vi "Create Control Custom Device.vi"(8 "error in (no error)":errorcluster, 9 "CD Config Path (.dat)":path, 10 "Name":string, 11 "Custom Devices Ref":refnum<k24>) -> (0 "error out":errorcluster, 3 "Custom Devices Ref":refnum<k24>)   [LabVIEW 2019, in "Control System Definition API.lvlib"]
uses:
  Control System Definition API.lvlib
  NationalInstruments.VeriStand.SystemDefinitionAPI
  Shared/Constants.vi
  <vilib>/NI/NI VeriStand Custom Device Import and Export Tool/ImportExport.lvlib
  Shared/Control Addon Shared.lvlib
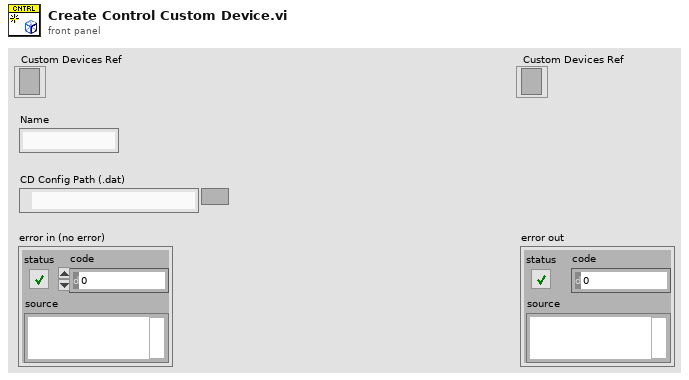
[diagram p1: front panel]
types:
  T1 = typedef "Custom Device API.lvlib/Custom Device Item Ref.ctl" = u64
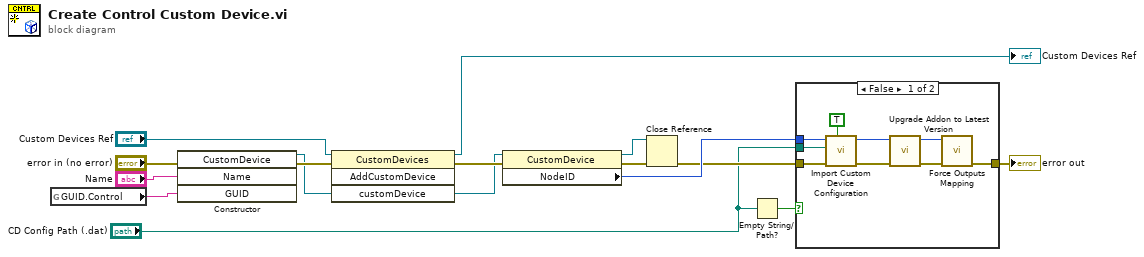
[diagram p0: block diagram]
diagram:
  n1 = global read "Constants.vi" "GUID.Control"() -> (w2:string)
  n2 = constructor class="CustomDevice"(error in="error in (no error)", "Name"="Name", "GUID"=w2) -> (reference out=w8:refnum<k24>, error out=w10:errorcluster)  [unwired: 2 in, 3 out]
  n3 = invoke class="CustomDevices" method="AddCustomDevice"(reference="Custom Devices Ref", error in=w10, "customDevice"=w8) -> (reference out=→"Custom Devices Ref":refnum<k24>, error out=w9:errorcluster)  [unwired: 1 in, 2 out]
  n4 = property class="CustomDevice"(reference=w8, error in=w9) -> (reference out=w7:refnum<k24>, error out=w6:errorcluster, "NodeID"=w13:u64)
  n5 = Close Reference(reference=w7, error in (no error)=w6) -> (error out=w5:errorcluster)
  n6 = Empty String/Path?(string/path="CD Config Path (.dat)") -> (empty?=w3:bool)
  n7 = case shown="False" w3 {
    tunnel: w13 -> [w24 _]
    tunnel: [w17 w25] -> w12
    tunnel: w5 -> [w22 w25]
    tunnel: "CD Config Path (.dat)" -> [w21 _]
    frame False {
      n8 = call <vilib>:"Import Custom Device Configuration.vi"("Overwrite Existing?"=TRUE, "error in (no error)"=w22, "Path"=w21, "NodeID"=w24) -> ("error out"=w20:errorcluster, "NodeID out"=w19:u64)  [unwired: 5 in, 1 out]
      n9 = call "Upgrade Addon to Latest Version.vi"("error in (no error)"=w20, "Device Item Ref in in"=w19) -> ("error out"=w16:errorcluster, "Device Item Ref out"=w18:T1)  [unwired: 8 in]
      n10 = call "Force Outputs Mapping.vi"("error in (no error)"=w16, "Device Item Ref in"=w18) -> ("error out"=w17:errorcluster)  [unwired: 8 in, 1 out]
    }
    frame True {
    }
  }
  "error out" <- w12
